vi "GetVersion.vi"(0 "controller in":refnum<k24>, 11 "error in (no error)":errorcluster) -> (4 "controller out":refnum<k24>, 6 "SMC version":string, 15 "error out":errorcluster)   [LabVIEW 2016, in "Aerotech VIs.lvlib"]
uses:
  Aerotech VIs.lvlib
  C:/Users/HEP Gantry/Documents/Assembly/V4/Drivers/Aerotech A3200/Bin/Aerotech.A3200.dll
  V4/Drivers/Aerotech A3200/Bin/Aerotech.A3200.dll
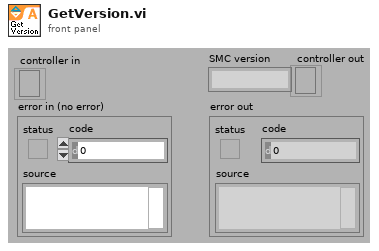
[diagram p1: front panel]
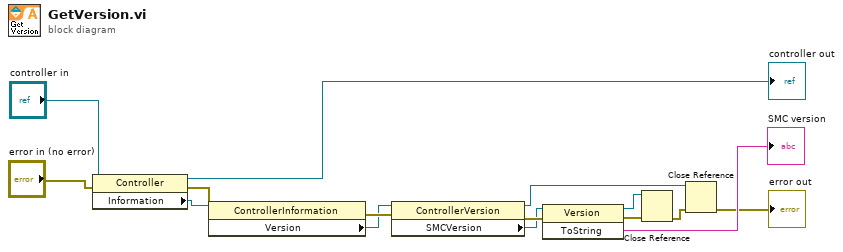
[diagram p0: block diagram]
diagram:
  n1 = property class="Controller"(reference="controller in", error in="error in (no error)") -> (reference out=→"controller out":refnum<k24>, error out=w3:errorcluster, "Information"=w7:refnum<k24>)
  n2 = property class="ControllerInformation"(reference=w7, error in=w3) -> (error out=w2:errorcluster, "Version"=w1:refnum<k24>)  [unwired: 1 out]
  n3 = property class="ControllerVersion"(reference=w1, error in=w2) -> (reference out=w10:refnum<k24>, error out=w12:errorcluster, "SMCVersion"=w8:refnum<k24>)
  n4 = invoke class="Version" method="ToString"(reference=w8, error in=w12) -> (reference out=w4:refnum<k24>, error out=w6:errorcluster, "ToString"=→"SMC version":string)  [unwired: 1 in]
  n5 = Close Reference(reference=w4, error in (no error)=w6) -> (error out=w5:errorcluster)
  n6 = Close Reference(reference=w10, error in (no error)=w5) -> (error out=→"error out":errorcluster)
